vi "Test Create Empty Set.vi"() -> ()   [LabVIEW 2020]
uses:
  8fec0cc0-9b33-44ff-9dc9-b4ec2d503673.vi
  <vilib>/addons/_JKI Toolkits/Caraya/classes/Assert/Assert Equal Value and Type_Variant.vi
  <vilib>/addons/_JKI Toolkits/Caraya/classes/Test/Test.lvclass
  <vilib>/addons/_JKI Toolkits/Caraya/classes/Assert/Assert.lvclass
panel:
  out "error out":errorcluster
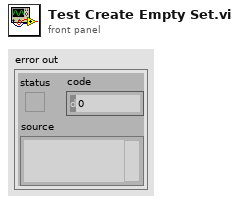
[diagram p1: front panel]
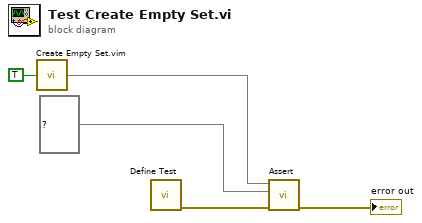
[diagram p0: block diagram]
diagram:
  n1 = call "Create Empty Set.vim"("element type"=TRUE) -> ("empty set"=w2:set{bool})  [unwired: 6 in]
  n2 = call <vilib>:"Define Test.vi"() -> ("error out"=w4:errorcluster)  [unwired: 11 in]
  n3 = call-poly <vilib>:"Assert.vi"("error in (no error)"=w4, "Y"=set{bool} {} ("empty set"), "X"=w2) -> ("error out"=→"error out":errorcluster)  [unwired: 8 in]
